vi "Process-received-message.vi"(8 "error in (no error)":errorcluster, 10 "Message":refnum<class "Message.lvclass">, 11 "Client in":T2) -> (0 "error out":errorcluster, 1 "Action":T1=enum."Initialize", 3 "Client out":T2)   [LabVIEW 2013, in "SLMControl.lvlib" / "SC-Client.lvclass"]
doc: "This function wraps the message checks, analysis and response action functions.\nThe validity of the message and message origin is checked, after which the appropriate module action is determined and executed.\n\nThe actions should be implemented by the module integrator."
uses:
  SC-Client.lvclass
  Object-reference.ctl
  SA-SLMAPI/Sources/Message.lvclass
  Supported-actions.ctl
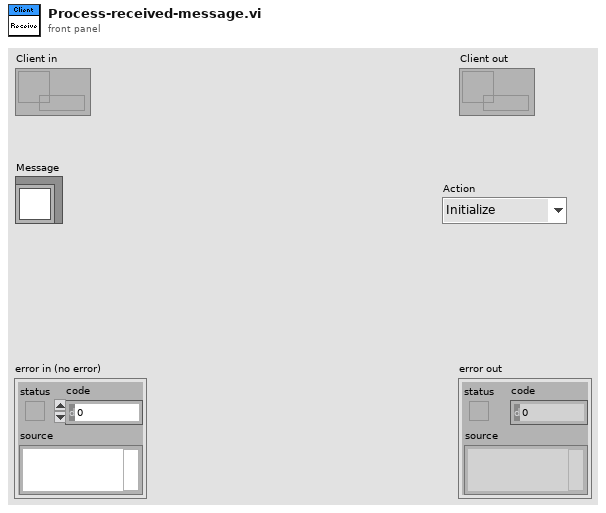
[diagram p1: front panel]
types:
  T1 = typedef "SLMControl.lvlib/SC-Client.lvclass/Supported-actions.ctl" = enum16{"Idle", "Initialize", "Load settings", "Load file", "Activate", "Start", "Pause", "Stop", "Repeat", "Reset", "Exit"}
  T2 = typedef "SLMControl.lvlib/SC-Client.lvclass/Object-reference.ctl" = refnum<data-value>
  T3 = typedef "SLMControl.lvlib/SC-Client.lvclass/Supported-messages.ctl" = enum16{"Heartbeat", "Error", "Start client", "Client stopped", "Action", "Query status", "Send status", "Get clients"}
  T4 = typedef "SLMControl.lvlib/SC-Client.lvclass/Supported-modules.ctl" = enum16{"Server", "All", "SLMControl", "PowderDeposition", "StrategyParser", "CameraVision", "MaterialCharacterization", "StatusMonitor", "SLMSimulation", "LaserCharacterization"}
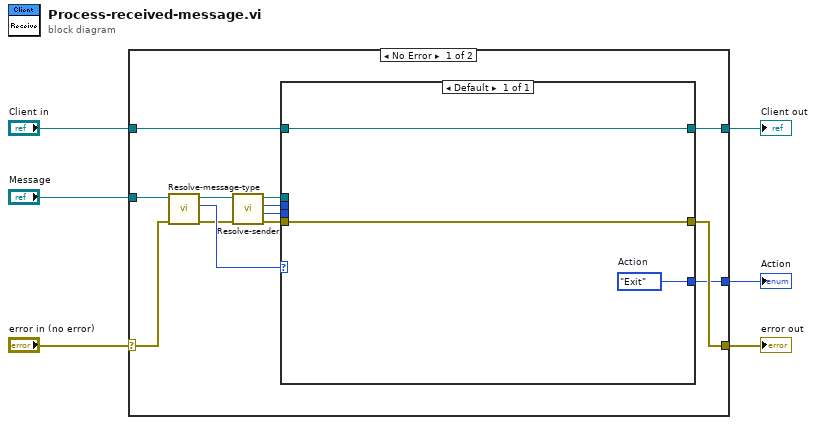
[diagram p0: block diagram]
diagram:
  n1 = case shown="No Error" "error in (no error)" {
    selector: "error in (no error)" -> [w16 w24]
    tunnel: [w19 w24] -> w5
    tunnel: [w17 w23] -> w3
    tunnel: "Client in" -> [w18 w23]
    tunnel: "Message" -> [w15 _]
    tunnel: [w7 _] -> w1
    frame No Error {
      n2 = call "Resolve-message-type.vi"("error in (no error)"=w16, "Message"=w15) -> ("error out"=w12:errorcluster, "Message type"=w14:T3, "Message dup"=w13:refnum<class "Message.lvclass">)  [unwired: 7 in]
      n3 = call "Resolve-sender.vi"("error in (no error)"=w12, "Message"=w13) -> ("error out"=w9:errorcluster, "Sender ID"=w10:i32, "Sender type"=w11:T4, "Message dup"=w8:refnum<class "Message.lvclass">)  [unwired: 6 in]
      n4 = case shown="Default" w14 {
        tunnel: [w21] -> w19
        tunnel: w18 -> [w22]
        tunnel: [w22] -> w17
        tunnel: w11 -> [_]
        tunnel: w10 -> [_]
        tunnel: w9 -> [w21]
        tunnel: w8 -> [_]
        tunnel: [w20] -> w7
        frame Default {
          w20 = Supported-actions."Exit"  # Action
        }
      }
    }
    frame Error {
    }
  }
  "error out" <- w5
  "Client out" <- w3
  "Action" <- w1
